vi "set_point_package_size.vi"(8 "error in (no error)":errorcluster, 10 "point package size":u8, 11 "FPGAWrapperMH120124RAPS_PXI7813R in":refnum<class "FPGAWrapperMH120124RAPS_PXI7813R.lvclass">) -> (0 "error out":errorcluster, 3 "FPGAWrapperMH120124RAPS_PXI7813R out":refnum<class "FPGAWrapperMH120124RAPS_PXI7813R.lvclass">)   [LabVIEW 2010, in "FPGAWrapperMH120124RAPS_PXI7813R.lvclass"]
uses:
  FPGAWrapperMH120124RAPS_PXI7813R.lvclass
  FPGAWrapperMH120124RAPS_PXI7813R.lvclass/FPGAWrapperMH120124RAPS_PXI7813R.ctl
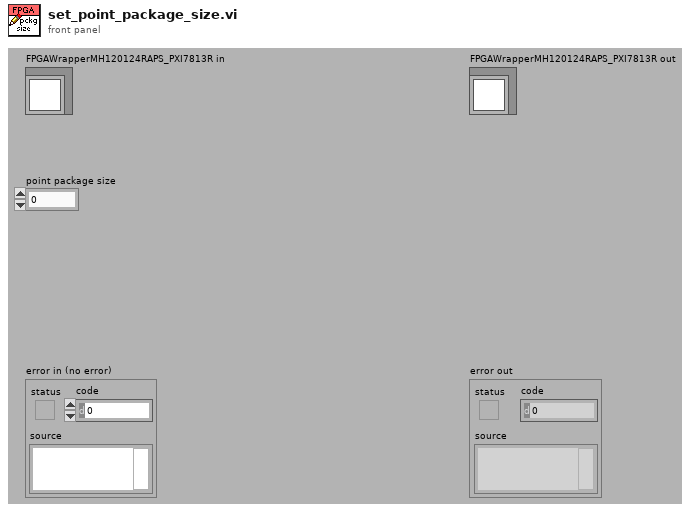
[diagram p1: front panel]
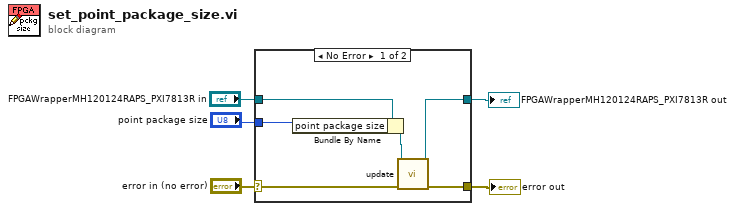
[diagram p0: block diagram]
diagram:
  n1 = case shown="No Error" "error in (no error)" {
    selector: "error in (no error)" -> [w7 w13]
    tunnel: [w6 w13] -> w4
    tunnel: [w8 w12] -> w2
    tunnel: "FPGAWrapperMH120124RAPS_PXI7813R in" -> [w9 w12]
    tunnel: "point package size" -> [w11 _]
    frame No Error {
      n2 = Bundle By Name(cluster=w9, "point package size"=w11) -> (w10:refnum<class "FPGAWrapperMH120124RAPS_PXI7813R.lvclass">)
      n3 = call-dynamic "update.vi"("error in (no error)"=w7, "FPGAWrapperMH120124RAPS_PXI7813R in"=w10) -> ("error out"=w6:errorcluster, "FPGAWrapperMH120124RAPS_PXI7813R out"=w8:refnum<class "FPGAWrapperMH120124RAPS_PXI7813R.lvclass">)  [unwired: 8 in]
    }
    frame Error {
    }
  }
  "error out" <- w4
  "FPGAWrapperMH120124RAPS_PXI7813R out" <- w2
